vi "Stop Beacon.vi"   [LabVIEW 2020, in "epl-network.lvlib"]
uses:
  epl-network.lvlib
  afc993c7-4e33-4e74-80a4-61b5b983949b.vi
types:
  T1 = typedef "epl-network.lvlib/Beacon FGV.ctl" = cluster{"receiver":refnum<vi>, "stop":refnum<notifier>}
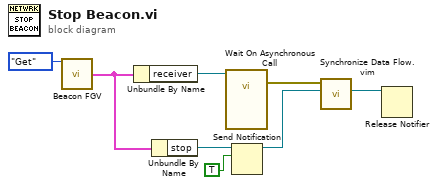
[diagram p0: block diagram]
diagram:
  n1 = call "Beacon FGV.vi"("action"=enum16{"Initialize", "Get"}."Get") -> ("data out"=w2:T1)  [unwired: 14 in]
  n2 = Unbundle By Name(w2) -> ("receiver"=w3:refnum<vi>)
  n3 = Unbundle By Name(w2) -> ("stop"=w6:refnum<notifier>)
  n4 = call-by-ref "Wait On Asynchronous Call"(reference=w3) -> (error out=w1:errorcluster)  [unwired: 17 in, 1 out]
  n5 = Send Notification(notification=TRUE, notifier=w6) -> (notifier out=w5:refnum<notifier>)  [unwired: 1 in, 1 out]
  n6 = call "Synchronize Data Flow.vim"("input 2"=w5, "input 1"=w1) -> ("output 2"=w4:refnum<notifier>)  [unwired: 2 in, 3 out]
  n7 = Release Notifier(notifier=w4) -> ()  [unwired: 2 in, 3 out]
